vi "836_CameraGet Image From Controller.vi"(4 "Camera Settings":T1={"fps"=30, "compression"=30, "Image Size"=enum."320x240"}, 6 "USB":bool, 7 "Camera Mode":u16(ring) items=["Camera Off", "USB Camera SW", "USB Camera HW", "IP Camera"], 8 "error in (no error)":errorcluster, 9 "Close?":bool, 10 "Controller Address":string, 11 "Image":T3) -> (0 "error out":errorcluster, 2 "Bandwidth (Mbps)":dbl=30.0, 3 "Image Out":T3(plugin-control))   [LabVIEW 2015]
doc: "Retrieves a specific image from the image data that the camera connected to the CompactRIO device you specify acquired. Use this VI in the FRC dashboard project on the host computer.\n\nThis software is licensed. Open the labview\\readme\\WPI Robotics Library Open Source License.txt file for more information."
uses:
  <vilib>/vision/Image Controls.llb/IMAQ Image.ctl
  <vilib>/Rock Robotics/WPI/Camera/WPI_CameraSettings Read MJPG.ctl
  <vilib>/Rock Robotics/WPI/Camera/WPI_CameraImageSize.ctl
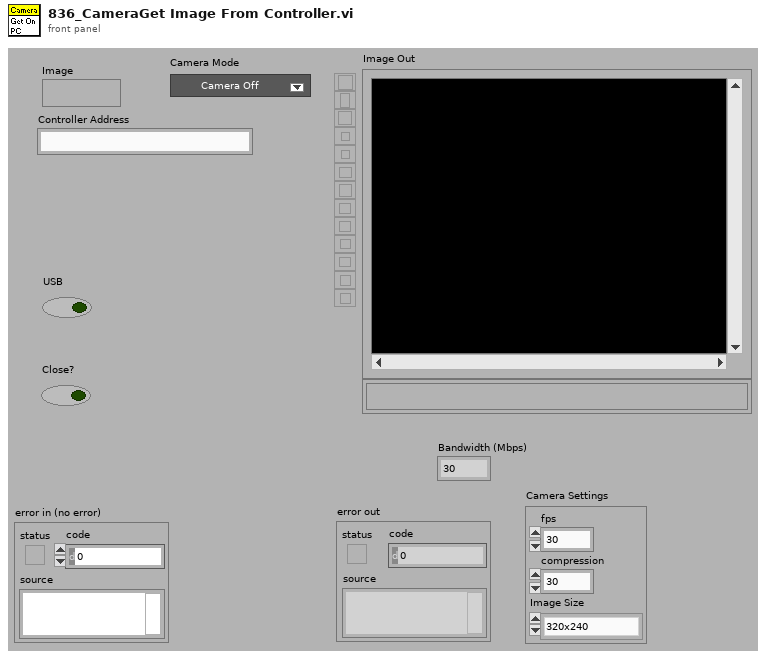
[diagram p1: front panel]
types:
  T1 = typedef "WPI_CameraSettings Read MJPG.ctl" = cluster{"fps":i32, "compression":i32, "Image Size":T2}
  T2 = typedef "WPI_CameraImageSize.ctl" = enum16{"640x480", "320x240", "160x120", "Custom"}
  T3 = typedef "IMAQ Image.ctl" = refnum<image>
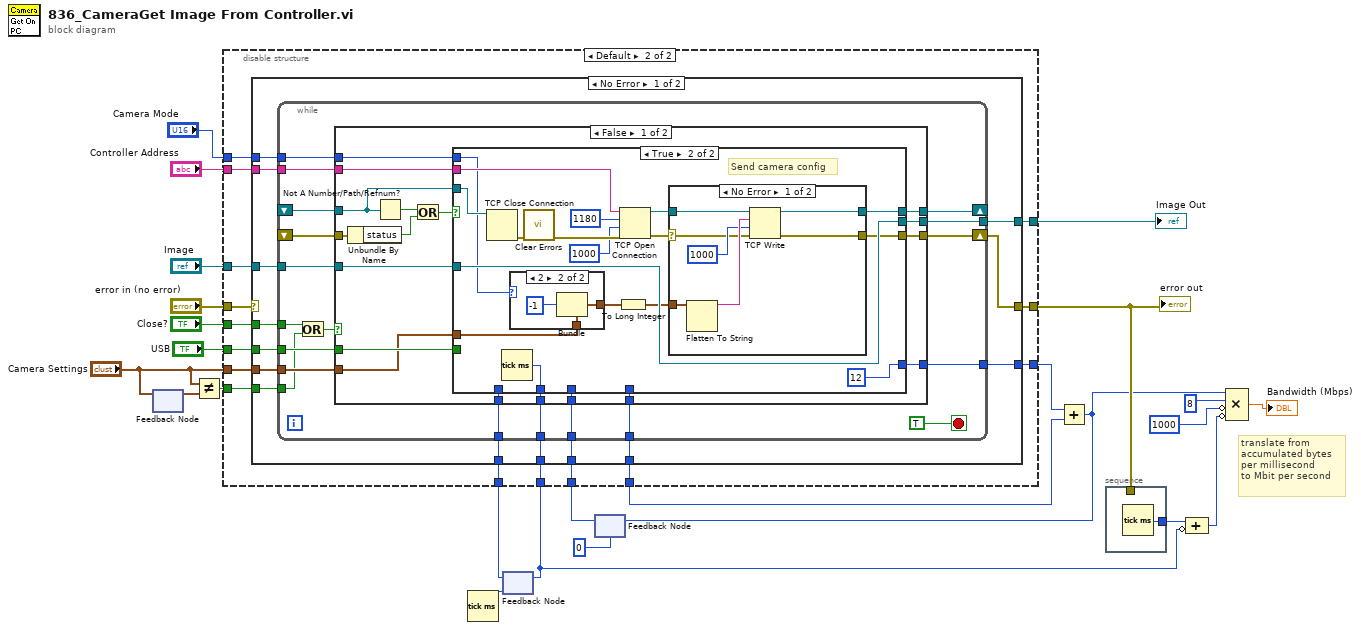
[diagram p0: block diagram]
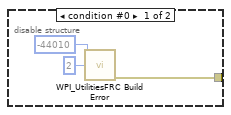
[diagram p2: hidden frame]
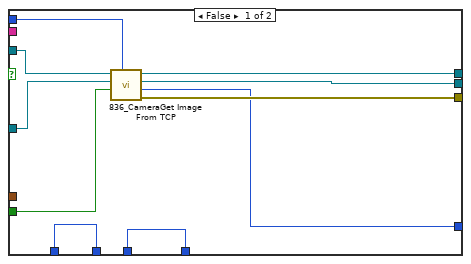
[diagram p3: hidden frame]
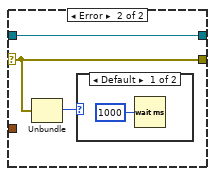
[diagram p5: hidden frame]
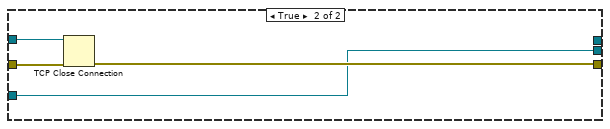
[diagram p7: hidden frame]
diagram:
  # "translate from\naccumulated bytes\nper millisecond \nto Mbit per second"
  n1 = feedback-in #1("Camera Settings") -> ()
  n2 = feedback #1() -> (w18:T1)  [unwired: 1 in]
  n3 = Not Equal?(x="Camera Settings", y=w18) -> (x != y?=w16:bool)
  n4 = Tick Count (ms)() -> (millisecond timer value=w15:u32)
  n5 = feedback #2(w15) -> (w5:u32)
  n6 = feedback #3(0) -> (w4:i32)
  n7 = disable-structure shown="Default" {
    disable-tunnel: "error in (no error)" -> [_ w42]
    disable-tunnel: [w25 w41] -> w8
    disable-tunnel: "Close?" -> [_ w40]
    disable-tunnel: "Image" -> [_ w39]
    disable-tunnel: [_ w38] -> w21
    disable-tunnel: "Controller Address" -> [_ w37]
    disable-tunnel: "USB" -> [_ w36]
    disable-tunnel: "Camera Settings" -> [_ w35]
    disable-tunnel: w16 -> [_ w34]
    disable-tunnel: [_ w33] -> w6
    disable-tunnel: w5 -> [_ w32]
    disable-tunnel: w4 -> [_ w31]
    disable-tunnel: [_ w30] -> w3
    disable-tunnel: [_ w29] -> w2
    disable-tunnel: "Camera Mode" -> [_ w28]
    frame condition #0 {
      n8 = call <vilib>:"WPI_UtilitiesFRC Build Error.vi"("error code"=-44010 ("code"), "chain levels to remove (1)"=2) -> ("error out"=w25:errorcluster)  [unwired: 3 in, 10 out]
    }
    frame condition #1 (active) {
      n9 = case shown="No Error" w42 {
        selector: w42 -> [_ w143]
        tunnel: [w56 w143] -> w41
        tunnel: w40 -> [w55 _]
        tunnel: w39 -> [w54 w142]
        tunnel: [w53 w142] -> w38
        tunnel: w37 -> [w52 _]
        tunnel: w36 -> [w51 _]
        tunnel: w35 -> [w50 _]
        tunnel: w34 -> [w49 _]
        tunnel: [w48 w141] -> w33
        tunnel: w32 -> [w47 w141]
        tunnel: w31 -> [w46 w140]
        tunnel: [w45 w140] -> w30
        tunnel: [w44 _] -> w29
        tunnel: w28 -> [w43 _]
        frame No Error {
          n10 = while {
            shift-right: [w75] -> w56
            shift-left: _ -> [w73]
            shift-right: [w74] -> _
            shift-left: _ -> [w72]
            tunnel: w55 -> [w65]
            tunnel: w54 -> [w70]
            tunnel: [w69] -> w53
            tunnel: w52 -> [w68]
            tunnel: w51 -> [w67]
            tunnel: w50 -> [w66]
            tunnel: w49 -> [w63]
            tunnel: [w62] -> w48
            tunnel: w47 -> [w61]
            tunnel: w46 -> [w60]
            tunnel: [w59] -> w45
            tunnel: [w58] -> w44
            tunnel: w43 -> [w57]
            stop <- TRUE stop-if-true
            n11 = Or(x=w65, y=w63) -> (x .or. y?=w64:bool)
            n12 = case shown="False" w64 {
              tunnel: [w93 w137] -> w75
              tunnel: [w92 _] -> w74
              tunnel: w73 -> [w91 w138]
              tunnel: w72 -> [w87 w139]
              tunnel: w70 -> [w86 w136]
              tunnel: [w85 w136] -> w69
              tunnel: w68 -> [w84 _]
              tunnel: w67 -> [w83 _]
              tunnel: w66 -> [w82 _]
              tunnel: [w81 _] -> w62
              tunnel: w61 -> [w80 _]
              tunnel: w60 -> [w79 _]
              tunnel: [w78 _] -> w59
              tunnel: [w77 _] -> w58
              tunnel: w57 -> [w76 _]
              frame False {
                n13 = Unbundle By Name(w91) -> ("status"=w89:bool)
                n14 = Not A Number/Path/Refnum?(number/path/refnum=w87) -> (NaN/Path/Refnum?=w90:bool)
                n15 = Or(x=w90, y=w89) -> (x .or. y?=w88:bool)
                n16 = case shown="True" w88 {
                  tunnel: [w103 w110] -> w93
                  tunnel: [w101 w111] -> w92
                  tunnel: w87 -> [w102 w120]
                  tunnel: w86 -> [w100 w116]
                  tunnel: [w99 w116] -> w85
                  tunnel: w84 -> [_ w115]
                  tunnel: w83 -> [w98 _]
                  tunnel: w82 -> [_ w106]
                  tunnel: [w97 w108] -> w81
                  tunnel: w80 -> [w97 _]
                  tunnel: w79 -> [w95 _]
                  tunnel: [w95 _] -> w78
                  tunnel: [w96 12 ("timeout ms (wait forever: -1)")] -> w77
                  tunnel: w76 -> [w94 w104]
                  frame False {
                    n17 = call "836_CameraGet Image From TCP.vi"("Camera Mode"=w94, "USB"=w98, "Image In"=w100, "connection ID"=w102) -> ("error out"=w103:errorcluster, "Size"=w96:i32, "Image Out"=w99:T3, "connection ID (dup)"=w101:refnum<k5>)  [unwired: 2 in, 2 out]
                  }
                  frame True {
                    # "Send camera config"
                    n18 = TCP Close Connection(connection ID=w120) -> (error out=w119:errorcluster)  [unwired: 1 in, 2 out]
                    n19 = Tick Count (ms)() -> (millisecond timer value=w108:u32)
                    n20 = case shown="2" w104 {
                      tunnel: w106 -> [w121 w124]
                      tunnel: [w121 w123] -> w105
                      frame 0, Default {
                      }
                      frame 2 {
                        n21 = Bundle(cluster=w124, "compression"=-1) -> (w123:T1)  [unwired: 2 in]
                      }
                    }
                    n22 = call <vilib>:"Clear Errors.vi"("error in (no error)"=w119) -> ("error out"=w118:errorcluster)  [unwired: 1 in, 5 out]
                    n23 = To Long Integer(number=w105) -> (32bit integer=w109:cluster{"fps":i32, "compression":i32, i32})
                    n24 = TCP Open Connection(address=w115, remote port or service name=u16 1180 ("port"), timeout ms (60000)=1000 ("timeout ms (wait forever: -1)"), error in (no error)=w118) -> (connection ID=w113:refnum<k5>, error out=w112:errorcluster)  [unwired: 1 out]
                    n25 = case shown="No Error" w112 {
                      selector: w112 -> [w125 w132]
                      tunnel: w113 -> [w131 w133]
                      tunnel: [w127 w133] -> w111
                      tunnel: [w126 w132] -> w110
                      tunnel: w109 -> [w130 _]
                      frame No Error {
                        n26 = Flatten To String(anything=w130) -> (data string=w129:string)  [unwired: 3 in, 2 out]
                        n27 = TCP Write(connection ID=w131, data in=w129, error in (no error)=w125, 9:1000 ("timeout ms (25000)")) -> (connection ID out=w127:refnum<k5>, error out=w126:errorcluster)  [unwired: 1 out]
                      }
                      frame Error {
                        n28 = Unbundle(w132) -> ("code"=w134:i32)  [unwired: 2 out]
                        n29 = case shown="Default" w134 {
                          frame Default {
                            n30 = Wait (ms)(milliseconds to wait=u32 1000) -> ()  [unwired: 1 out]
                          }
                          frame 56 {
                          }
                        }
                      }
                    }
                  }
                }
              }
              frame True {
                n31 = TCP Close Connection(connection ID=w139, error in (no error)=w138) -> (error out=w137:errorcluster)  [unwired: 2 out]
              }
            }
          }
        }
        frame Error {
        }
      }
    }
  }
  "error out" <- w8
  "Image Out" <- w21
  n32 = feedback-in #2(w6) -> ()
  n33 = Add(x=w2, y=w3) -> (x+y=w7:i32)
  n34 = feedback-in #3(w7) -> ()
  n35 = stacked-sequence {
    tunnel: [w144] -> w11
    tunnel: w8 -> [_]
    frame #0 {
      n36 = Tick Count (ms)() -> (millisecond timer value=w144:u32)
    }
  }
  n37 = Compound Arithmetic op=ADD(w11, invert w6) -> (w12:u32)
  n38 = Compound Arithmetic op=MULTIPLY(w7, 8 ("timeout ms (25000)"), invert 1000 ("timeout ms (25000)"), invert w12) -> (→"Bandwidth (Mbps)":dbl)
